vi "OAT Get Even Angle Signal Subset..vi"(0 "even angle signals (x-y)":cluster{"r0":dbl, "dr":dbl, "Y":dbl[]}[](array[cluster]) {"r0" format="%.2p"; "dr" format="%.2p"; "Y" format="%.2f"}, 5 "even angle channel info":T1[](array[typedef])=[{"channel name"="", "description"="", " channel info"={"sensor sensitivity [mV/EU]"=1000.0, "engineering units"=0, "dB reference [EU]"=1.0, "custom label"="EU", "weighting filter"=0, "pregain [dB]"=0.0}}, {"channel name"="", "description"="", " channel info"={"sensor sensitivity [mV/EU]"=1000.0, "engineering units"=0, "dB reference [EU]"=1.0, "custom label"="EU", "weighting filter"=0, "pregain [dB]"=0.0}}] {"channel info"."pregain [dB]" format="%.2f"; "channel info"."weighting filter" items=["Linear", "A-weighting", "B-weighting", "C-weighting", "ITU-R 468-4", "Dolby", "CCITT", "C-message"]; "channel info"."dB reference [EU]" format="%^.1e"; "channel info"."engineering units" items=["custom..."=0, "V"=1, "A"=21, "Pa"=2, "N"=20, "g"=3, "m/s^2"=4, "m/s"=5, "m"=6, "mm/s"=12, "mm"=13, "microns/s"=14, "microns"=15, "in/s^2"=7, "in/s"=8, "in"=9, "mils/s"=10, "mils"=11, "rad/s^2"=16, "rad/s"=17, "rad"=18, "strain"=19]; "channel info"."sensor sensitivity [mV/EU]" format="%.2f"}, 7 "revolution subset [rev]":cluster{"start":dbl, "duration":dbl}={"start"=0.0, "duration"=1.0} {"duration" format="%.2f"; "start" format="%.2f"}, 11 "error in (no error)":errorcluster) -> (4 "even angle signals (x-y) out":cluster{"r0":dbl, "dr":dbl, "Y":dbl[]}[](array[cluster]) {"r0" format="%.2p"; "dr" format="%.2p"; "Y" format="%.2f"}, 6 "dup even angle channel info":T1[](array[typedef])=[{"channel name"="", "description"="", " channel info"={"sensor sensitivity [mV/EU]"=1000.0, "engineering units"=0, "dB reference [EU]"=1.0, "custom label"="EU", "weighting filter"=0, "pregain [dB]"=0.0}}, {"channel name"="", "description"="", " channel info"={"sensor sensitivity [mV/EU]"=1000.0, "engineering units"=0, "dB reference [EU]"=1.0, "custom label"="EU", "weighting filter"=0, "pregain [dB]"=0.0}}] {"channel info"."pregain [dB]" format="%.2f"; "channel info"."weighting filter" items=["Linear", "A-weighting", "B-weighting", "C-weighting", "ITU-R 468-4", "Dolby", "CCITT", "C-message"]; "channel info"."dB reference [EU]" format="%^.1e"; "channel info"."engineering units" items=["custom..."=0, "V"=1, "A"=21, "Pa"=2, "N"=20, "g"=3, "m/s^2"=4, "m/s"=5, "m"=6, "mm/s"=12, "mm"=13, "microns/s"=14, "microns"=15, "in/s^2"=7, "in/s"=8, "in"=9, "mils/s"=10, "mils"=11, "rad/s^2"=16, "rad/s"=17, "rad"=18, "strain"=19]; "channel info"."sensor sensitivity [mV/EU]" format="%.2f"}, 15 "error out":errorcluster)   [LabVIEW 2012]
uses:
  <vilib>/addons/Sound and Vibration/compatibility/Controls/svl_Resampled Channel Info.ctl
  <vilib>/addons/Sound and Vibration/compatibility/Controls/svl_Channel Info.ctl
  <vilib>/addons/Sound and Vibration/compatibility/Controls/svl_Engineering Units Text Ring.ctl
  <vilib>/addons/Sound and Vibration/compatibility/Controls/svl_Weighting Filter Text Ring.ctl
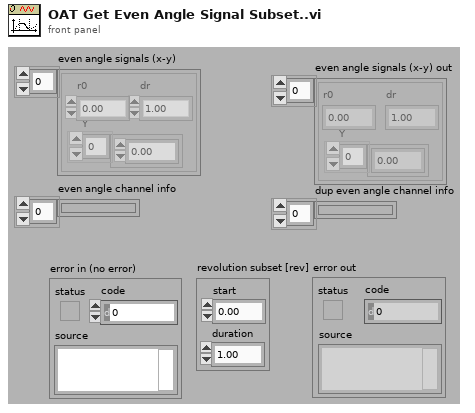
[diagram p1: front panel]
types:
  T1 = typedef "svl_Resampled Channel Info.ctl" = cluster{"channel name":string, "description":string, " channel info":T2}
  T2 = typedef "svl_Channel Info.ctl" = cluster{"sensor sensitivity [mV/EU]":dbl, "engineering units":T3, "dB reference [EU]":dbl, "custom label":string, "weighting filter":T4, "pregain [dB]":dbl}
  T3 = typedef "svl_Engineering Units Text Ring.ctl" = u16
  T4 = typedef "svl_Weighting Filter Text Ring.ctl" = u16
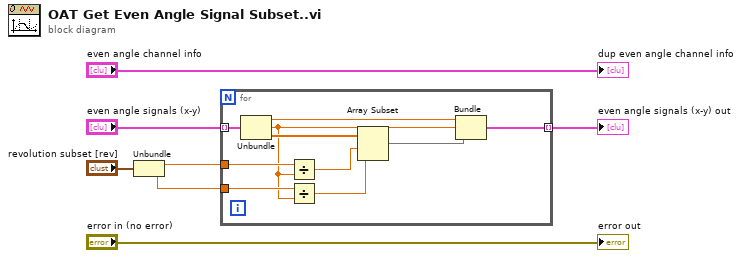
[diagram p0: block diagram]
diagram:
  n1 = Unbundle("revolution subset [rev]") -> ("start"=w4:dbl, "duration"=w3:dbl)
  n2 = for {
    tunnel: "even angle signals (x-y)" -> [w17] mode=indexing
    tunnel: w4 -> [w16]
    tunnel: w3 -> [w15]
    tunnel: [w8] -> w2 mode=indexing
    n3 = Unbundle(w17) -> ("r0"=w11:dbl, "dr"=w10:dbl, "Y"=w14:dbl[])
    n4 = Divide(x=w16, y=w10) -> (x/y=w13:dbl)
    n5 = Divide(x=w15, y=w10) -> (x/y=w12:dbl)
    n6 = Array Subset(array=w14, index=w13, length=w12) -> (w9:dbl[])
    n7 = Bundle("r0"=w11, "dr"=w10, w9) -> (w8:cluster{"r0":dbl, "dr":dbl, dbl[]})  [unwired: 1 out]
  }
  "even angle signals (x-y) out" <- w2
  "error out" <- "error in (no error)"
  "dup even angle channel info" <- "even angle channel info"
